vi "run.vi"(8 "error in (no error)":errorcluster, 11 "DL090324Microscope in":refnum<class "InstrumentDL090324.lvclass">) -> (0 "error out":errorcluster, 3 "DL090324Microscope out":refnum<class "InstrumentDL090324.lvclass">)   [LabVIEW 2010, in "InstrumentDL090324.lvclass"]
uses:
  InstrumentDL090324.lvclass
  internal_trigger_enum.ctl
  main/labview_source/controls/undock_button.ctl
  InstrumentDL090324.lvclass/InstrumentDL090324.ctl
  GenericInstrument/GenericInstrument/GenericInstrument.lvclass
  Detector/GenericDetector/GenericDetector/GenericDetector.lvclass
  LightSource/GenericLightSource/GenericLightSource/GenericLightSource.lvclass
  common/classes/ErrorController/ErrorController/class_data.vi
  common/classes/ErrorController/ErrorController/ErrorController.lvclass
panel:
  in  "button:undock":T1
  in  "Tab Control":enum32{"User", "Debug", "About"}(tab)
  in  "adjust buttons light source":bool[](array[boolean])
  in  "adjust buttons detectors":bool[](array[boolean])
  out "last trigger":T2
  out "statechart\nerror":errorcluster
  out "finished?":bool
  out "stache machine counter":i32
  # "Detectors"
  # "Light source"
  # "InstrumentDL090324\n\nImplemented by:\n- Dominik Langer, University of Zurich, Switzerland\n- Marcel van 't Hoff, University of Zurich, Switzerland"
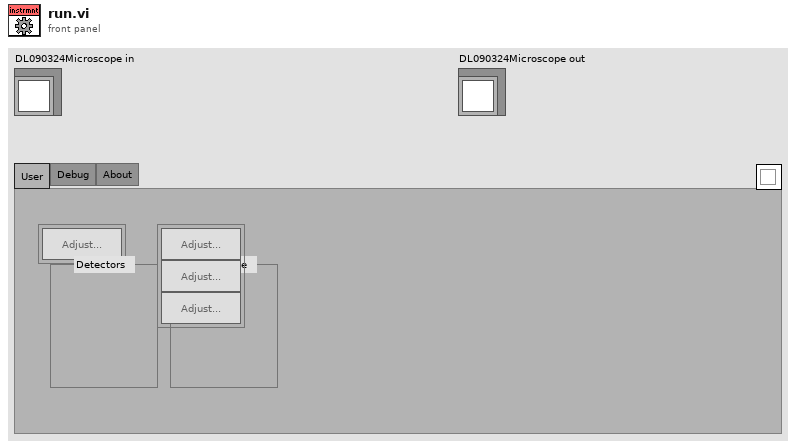
[diagram p1: front panel]
types:
  T1 = typedef "undock_button.ctl" = bool
  T2 = typedef "InstrumentDL090324.lvclass/internal_trigger_enum.ctl" = enum16{"NULL", "initialise", "terminate", "start", "stop"}
  T3 = typedef "top-level_component_type_enum.ctl" = enum16{"undefined", "ImagingMode", "ScanHead", "DAQ", "ImageAssembler", "Display", "DataCollection", "Analyser", "Stimulator", "ExperimentController", "Instrument", "Stage"}
  T4 = typedef "main_trigger_enum.ctl" = enum16{"NULL", "initialise", "terminate", "start", "stop", "change objective", "change experimentController", "change imagingMode", "save notebook", "started saving", "finished saving", "expCtr ready", "expCtr missing", "imgMd ready", "imgMd missing", "scanHd ready", "scanHd missing", "DAQ ready", "DAQ missing", "imgAsm ready", "imgAsm missing", "dataColl ready", "dataColl missing", "display ready", "display missing", "analysr ready", "analysr missing", "instrmnt ready", "instrmnt missing", "stimltr ready", "stimltr missing", "stage ready", "stage missing"}
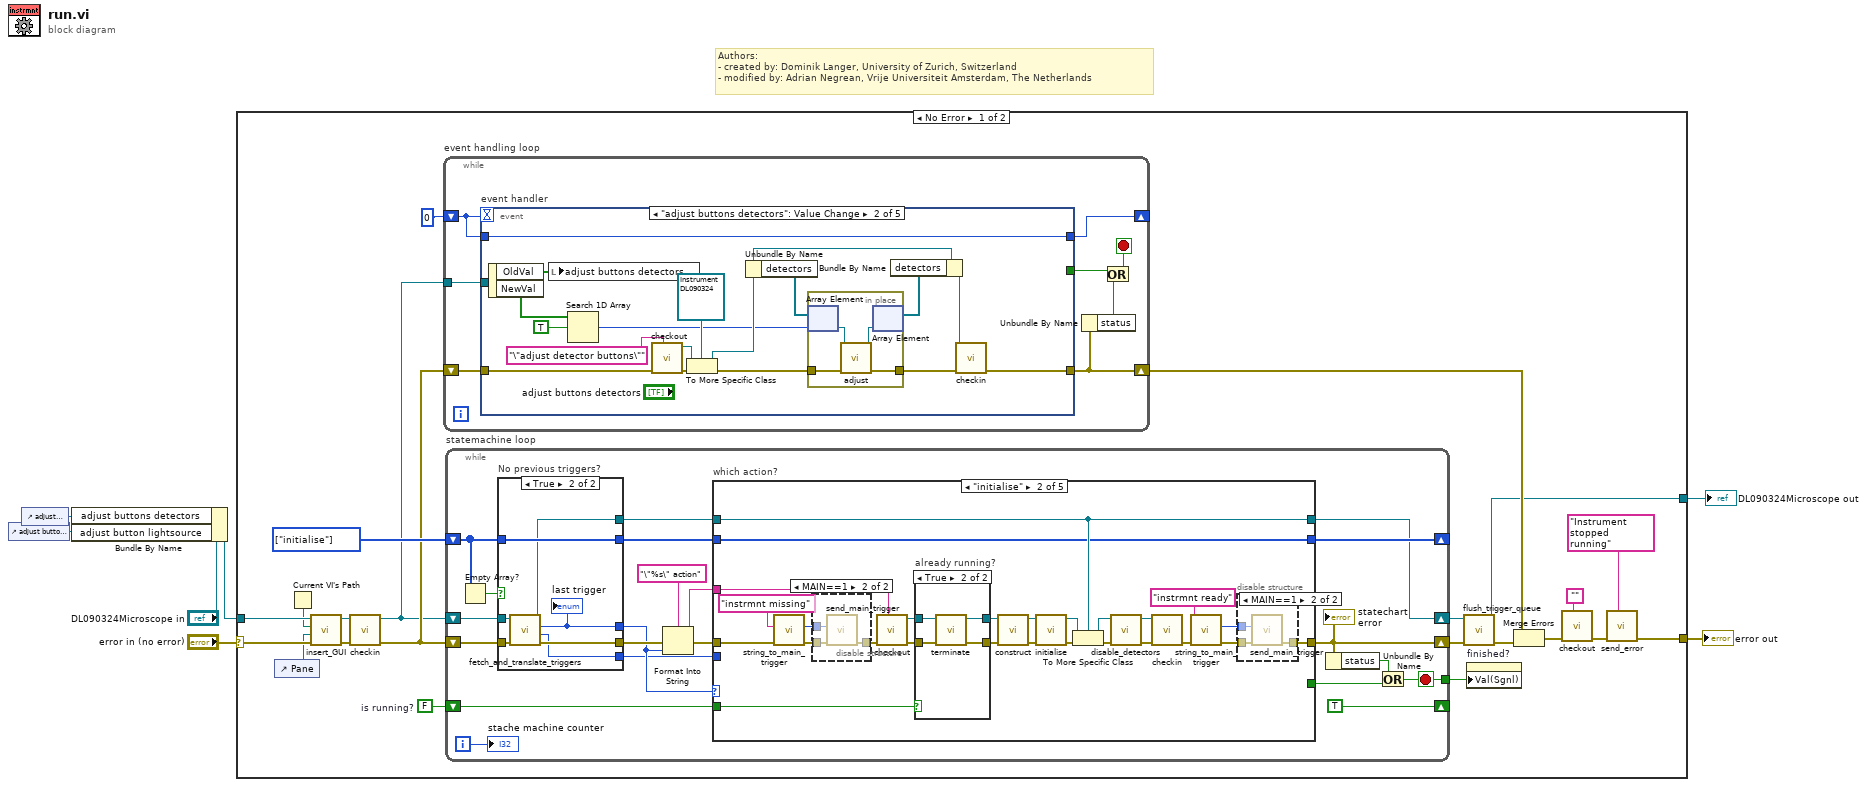
[diagram p0: block diagram]
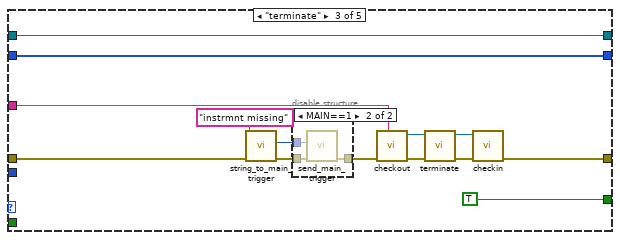
[diagram p6: hidden frame]
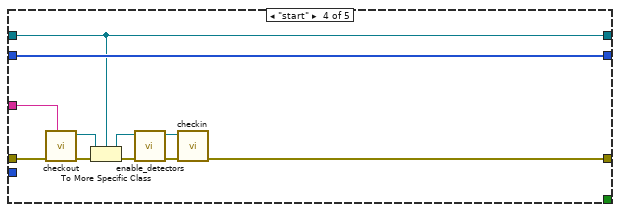
[diagram p8: hidden frame]
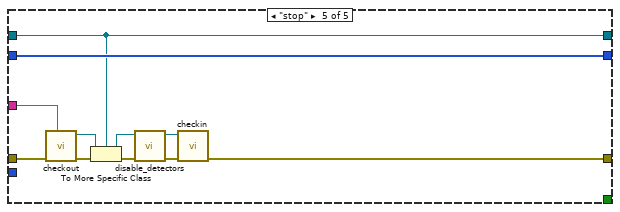
[diagram p9: hidden frame]
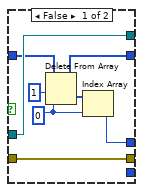
[diagram p10: hidden frame]
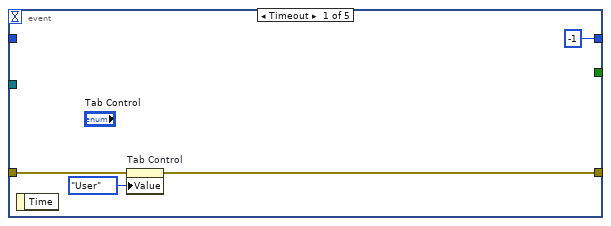
[diagram p11: hidden frame]
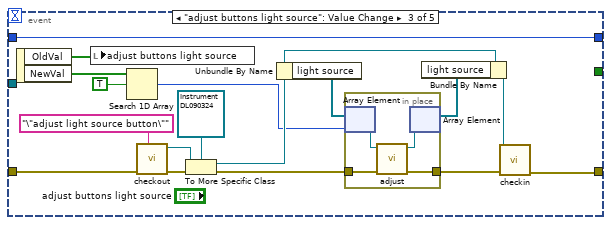
[diagram p12: hidden frame]
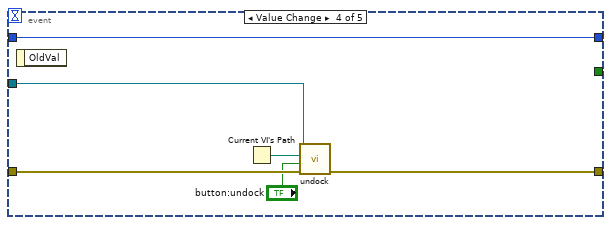
[diagram p13: hidden frame]
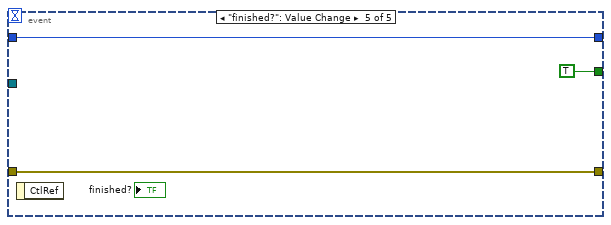
[diagram p14: hidden frame]
diagram:
  # "Authors: \n- created by: Dominik Langer, University of Zurich, Switzerland\n- modified by: Adrian Negrean, Vrije Universiteit Amsterdam, The Netherlands"
  n1 = control-ref of="adjust button lightsource"() -> (w1:refnum<vi>)
  n2 = control-ref of="adjust buttons detectors"() -> (w4:refnum<vi>)
  n3 = Bundle By Name(cluster="DL090324Microscope in", "adjust buttons detectors"=w4, "adjust button lightsource"=w1) -> (w2:refnum<class "InstrumentDL090324.lvclass">)
  n4 = case shown="No Error" "error in (no error)" {
    selector: "error in (no error)" -> [w27 w213]
    tunnel: [w22 w213] -> w6
    tunnel: [w12 w212] -> w5
    tunnel: w2 -> [w26 w212]
    frame No Error {
      w17 = FALSE  # is running?
      w18 = T2[] [enum."initialise"] items=["NULL", "initialise", "terminate", "start", "stop"]
      n5 = control-ref of="Pane"() -> (w24:refnum<vi>)
      n6 = Current VI's Path() -> (path=w25:path)
      n7 = call-dynamic "insert_GUI.vi"("error in (no error)"=w27, "Pane"=w24, "VI path"=w25, "GenericComponent in"=w26) -> ("error out"=w11:errorcluster, "GenericComponent out"=w19:refnum<class "InstrumentDL090324.lvclass">)  [unwired: 6 in]
      n8 = call-dynamic "checkin.vi"("error in (no error)"=w11, "GenericMicroscope in"=w19) -> ("error out"=w9:errorcluster, "GenericMicroscope out"=w8:refnum<class "InstrumentDL090324.lvclass">)  [unwired: 8 in]
      n9 = while "event handling loop" {
        shift-right: [w155] -> _
        shift-left: 0 -> [w156]
        shift-right: [w153] -> w13
        shift-left: w9 -> [w154]
        tunnel: w8 -> [w149]
        stop <- w152 stop-if-true
        n10 = event "event handler" shown="[1] \"adjust buttons detectors\": Value Change" {
          selector: _ -> [_ _ _ _ _]
          dyn-events: _ -> [_ _ _ _ _]
          timeout: w156 -> [_ _ _ _ _]
          tunnel: w156 -> [_ w177 w198 w208 w211]
          tunnel: [-1 w177 w198 w208 w211] -> w155
          tunnel: w154 -> [w158 w164 w197 w206 w210]
          tunnel: [w157 w172 w184 w205 w210] -> w153
          tunnel: [_ _ _ _ TRUE] -> w151
          tunnel: w149 -> [_ _ _ w207 _]
          event Timeout {
            n11 = event-data() -> ()  [unwired: 2 out]
            n12 = property on="Tab Control" class="TabCtl (strict)"(error in=w158, "Value"=enum32{"User", "Debug", "About"}."User" ("Tab Control")) -> (error out=w157:errorcluster)  [unwired: 1 in, 1 out]
          }
          event "adjust buttons detectors": Value Change {
            n13 = event-data() -> ("OldVal"=w175:bool[], "NewVal"=w169:bool[])  [unwired: 1 out]
            n14 = local write "adjust buttons detectors"(w175) -> ()
            n15 = Search 1D Array(1D array=w169, element=TRUE) -> (index of element=w167:i32)  [unwired: 1 out]
            n16 = call "checkout.vi"("locked by?"="\"adjust detector buttons\"", "error in (no error)"=w164) -> ("error out"=w161:errorcluster, "GenericMicroscope out"=w162:refnum<class "GenericInstrument.lvclass">)  [unwired: 8 out]
            n17 = To More Specific Class(target class=refnum<class "InstrumentDL090324.lvclass"> refnum ("DL090324Microscope.lvclass"), reference=w162, error in=w161) -> (specific class reference=w170:refnum<class "InstrumentDL090324.lvclass">, error out=w174:errorcluster)
            n18 = Unbundle By Name(w170) -> ("detectors"=w166:refnum<class "GenericDetector.lvclass">[])
            n19 = in-place {
              in-place-border: w174 -> [w181]
              in-place-border: [w178] -> w173
              n20 = in-place-array #1(w166, w167) -> (w180:refnum<class "GenericDetector.lvclass">)
              n21 = call-dynamic "adjust.vi"("error in (no error)"=w181, "GenericEmissionSensor in"=w180) -> ("error out"=w178:errorcluster, "GenericEmissionSensor out"=w179:refnum<class "GenericDetector.lvclass">)  [unwired: 8 out]
              n22 = in-place-array #1(w179) -> (w165:refnum<class "GenericDetector.lvclass">[])  [unwired: 1 out]
            }
            n23 = Bundle By Name(cluster=w170, "detectors"=w165) -> (w171:refnum<class "InstrumentDL090324.lvclass">)
            n24 = call-dynamic "checkin.vi"("error in (no error)"=w173, "GenericMicroscope in"=w171) -> ("error out"=w172:errorcluster)  [unwired: 8 in, 1 out]
          }
          event "adjust buttons light source": Value Change {
            n25 = event-data() -> ("OldVal"=w192:bool[], "NewVal"=w190:bool[])  [unwired: 1 out]
            n26 = local write "adjust buttons light source"(w192) -> ()
            n27 = Search 1D Array(1D array=w190, element=TRUE) -> (index of element=w182:i32)  [unwired: 1 out]
            n28 = call "checkout.vi"("locked by?"="\"adjust light source button\"", "error in (no error)"=w197) -> ("error out"=w196:errorcluster, "GenericMicroscope out"=w195:refnum<class "GenericInstrument.lvclass">)  [unwired: 8 out]
            n29 = To More Specific Class(target class=refnum<class "InstrumentDL090324.lvclass"> refnum ("DL090324Microscope.lvclass"), reference=w195, error in=w196) -> (specific class reference=w183:refnum<class "InstrumentDL090324.lvclass">, error out=w185:errorcluster)
            n30 = Unbundle By Name(w183) -> ("light source"=w187:refnum<class "GenericLightSource.lvclass">[])
            n31 = in-place {
              in-place-border: w185 -> [w202]
              in-place-border: [w201] -> w189
              n32 = in-place-array #2(w187, w182) -> (w200:refnum<class "GenericLightSource.lvclass">)
              n33 = call-dynamic "adjust.vi"("error in (no error)"=w202, "GenericLightSource in"=w200) -> ("error out"=w201:errorcluster, "GenericLightSource out"=w199:refnum<class "GenericLightSource.lvclass">)  [unwired: 8 in]
              n34 = in-place-array #2(w199) -> (w186:refnum<class "GenericLightSource.lvclass">[])  [unwired: 1 out]
            }
            n35 = Bundle By Name(cluster=w183, "light source"=w186) -> (w188:refnum<class "InstrumentDL090324.lvclass">)
            n36 = call-dynamic "checkin.vi"("error in (no error)"=w189, "GenericMicroscope in"=w188) -> ("error out"=w184:errorcluster)  [unwired: 8 in, 1 out]
          }
          event Value Change {
            n37 = event-data() -> ()  [unwired: 2 out]
            n38 = Current VI's Path() -> (path=w203:path)
            n39 = call-dynamic "undock.vi"("error in (no error)"=w206, "undock?"="button:undock", "VI path"=w203, "component in"=w207) -> ("error out"=w205:errorcluster)  [unwired: 6 in, 1 out]
          }
          event "finished?": Value Change {
            n40 = event-data() -> ()  [unwired: 2 out]
          }
        }
        n41 = Unbundle By Name(w153) -> ("status"=w150:bool)
        n42 = Or(x=w151, y=w150) -> (x .or. y?=w152:bool)
      }
      n43 = while "statemachine loop" {
        shift-right: [w34] -> w15
        shift-left: w9 -> [w50]
        shift-right: [w40] -> _
        shift-left: w18 -> [w48]
        shift-right: [w38] -> w14
        shift-left: w8 -> [w49]
        shift-right: [TRUE ("is running?")] -> _
        shift-left: w17 -> [w37]
        tunnel: [w31] -> w16
        i -> [w30]
        stop <- w31 stop-if-true
        n44 = Empty Array?(array=w48) -> (empty?=w47:bool)
        n45 = case "No previous triggers?" shown="True" w47 {
          tunnel: w49 -> [w141 w145]
          tunnel: w50 -> [w139 w147]
          tunnel: [w141 w144] -> w39
          tunnel: [w137 w143] -> w44
          tunnel: [_ w142] -> w43
          tunnel: [w139 w146] -> w46
          tunnel: w48 -> [w140 w148]
          tunnel: [w136 w148] -> w41
          frame False {
            w134 = 0 ("index")
            n46 = Delete From Array(array=w140, length=1, index=w134) -> (deleted portion=w138:T2[], array with subset deleted=w136:T2[])
            n47 = Index Array(array=w138, index=w134) -> (element=w137:T2)
          }
          frame True {
            n48 = call-dynamic "fetch_and_translate_triggers.vi"("error in (no error)"=w147, "InstrumentDL090324 in"=w145) -> ("error out"=w146:errorcluster, "sender TLC type"=w142:T3, "statechart trigger"=w143:T2, "InstrumentDL090324 out"=w144:refnum<class "InstrumentDL090324.lvclass">)  [unwired: 6 in]
            "last trigger" <- w143
          }
        }
        n49 = Format Into String(format string="\"%s\" action", error in=w46, w44) -> (resulting string=w35:string, error out=w42:errorcluster)  [unwired: 1 in]
        n50 = case "which action?" shown="\"initialise\"" w44 {
          tunnel: w43 -> [_ _ _ _ _]
          tunnel: w42 -> [w51 w56 w95 w121 w132]
          tunnel: w41 -> [w53 w63 w107 w122 w133]
          tunnel: [w53 w63 w107 w122 w133] -> w40
          tunnel: w39 -> [w52 w66 w106 w117 w128]
          tunnel: [w52 w66 w106 w117 w128] -> w38
          tunnel: [w51 w71 w103 w116 w127] -> w34
          tunnel: w37 -> [_ w79 _ _ _]
          tunnel: w35 -> [_ w76 w102 w120 w131]
          tunnel: [_ _ TRUE ("is running?") _ _] -> w32
          frame "NULL", Default {
          }
          frame "initialise" {
            n51 = call "string_to_main_trigger.vi"("error in (no error)"=w56, "trigger string"="instrmnt missing") -> ("error out"=w57:errorcluster, "main trigger"=w58:T4)  [unwired: 8 in]
            n52 = disable-structure shown="MAIN==1" {
              disable-tunnel: [w80 w82] -> w55
              disable-tunnel: w57 -> [w80 w83]
              disable-tunnel: w58 -> [_ w81]
              frame condition #0 (active) {
              }
              frame condition #1 {
                n53 = call "send_main_trigger.vi"("error in (no error)"=w83, "trigger"=w81) -> ("error out"=w82:errorcluster)  [unwired: 9 in]
              }
            }
            n54 = call "checkout.vi"("locked by?"=w76, "error in (no error)"=w55) -> ("error out"=w78:errorcluster, "GenericMicroscope out"=w77:refnum<class "GenericInstrument.lvclass">)  [unwired: 8 out]
            n55 = case "already running?" shown="True" w79 {
              tunnel: w78 -> [w88 w93]
              tunnel: w77 -> [w89 w91]
              tunnel: [w88 w92] -> w75
              tunnel: [w89 w90] -> w74
              frame False {
              }
              frame True {
                n56 = call-dynamic "terminate.vi"("error in (no error)"=w93, "GenericPlugin in"=w91) -> ("error out"=w92:errorcluster, "GenericPlugin out"=w90:refnum<class "GenericInstrument.lvclass">)  [unwired: 8 out]
              }
            }
            n57 = call-dynamic "construct.vi"("error in (no error)"=w75, "GenericPlugin in"=w74) -> ("error out"=w72:errorcluster, "GenericPlugin out"=w73:refnum<class "GenericInstrument.lvclass">)  [unwired: 2 in, 6 out]
            n58 = call-dynamic "initialise.vi"("error in (no error)"=w72, "GenericPlugin in"=w73) -> ("error out"=w68:errorcluster, "GenericPlugin out"=w65:refnum<class "GenericInstrument.lvclass">)  [unwired: 8 in]
            n59 = To More Specific Class(target class=w66, reference=w65, error in=w68) -> (specific class reference=w64:refnum<class "InstrumentDL090324.lvclass">, error out=w67:errorcluster)
            n60 = call-dynamic "disable_detectors.vi"("error in (no error)"=w67, "DL090324Microscope in"=w64) -> ("error out"=w70:errorcluster, "DL090324Microscope out"=w69:refnum<class "InstrumentDL090324.lvclass">)  [unwired: 8 out]
            n61 = call-dynamic "checkin.vi"("error in (no error)"=w70, "GenericMicroscope in"=w69) -> ("error out"=w61:errorcluster)  [unwired: 8 in, 1 out]
            n62 = call "string_to_main_trigger.vi"("error in (no error)"=w61, "trigger string"="instrmnt ready") -> ("error out"=w60:errorcluster, "main trigger"=w59:T4)  [unwired: 8 in]
            n63 = disable-structure shown="MAIN==1" {
              disable-tunnel: [w84 w86] -> w71
              disable-tunnel: w60 -> [w84 w87]
              disable-tunnel: w59 -> [_ w85]
              frame condition #0 (active) {
              }
              frame condition #1 {
                n64 = call "send_main_trigger.vi"("error in (no error)"=w87, "trigger"=w85) -> ("error out"=w86:errorcluster)  [unwired: 9 in]
              }
            }
          }
          frame "terminate" {
            n65 = call "string_to_main_trigger.vi"("error in (no error)"=w95, "trigger string"="instrmnt missing") -> ("error out"=w97:errorcluster, "main trigger"=w96:T4)  [unwired: 8 in]
            n66 = disable-structure shown="MAIN==1" {
              disable-tunnel: [w108 w110] -> w94
              disable-tunnel: w97 -> [w108 w111]
              disable-tunnel: w96 -> [_ w109]
              frame condition #0 (active) {
              }
              frame condition #1 {
                n67 = call "send_main_trigger.vi"("error in (no error)"=w111, "trigger"=w109) -> ("error out"=w110:errorcluster)  [unwired: 9 in]
              }
            }
            n68 = call "checkout.vi"("locked by?"=w102, "error in (no error)"=w94) -> ("error out"=w105:errorcluster, "GenericMicroscope out"=w101:refnum<class "GenericInstrument.lvclass">)  [unwired: 8 out]
            n69 = call-dynamic "terminate.vi"("error in (no error)"=w105, "GenericPlugin in"=w101) -> ("error out"=w104:errorcluster, "GenericPlugin out"=w100:refnum<class "GenericInstrument.lvclass">)  [unwired: 8 out]
            n70 = call-dynamic "checkin.vi"("error in (no error)"=w104, "GenericMicroscope in"=w100) -> ("error out"=w103:errorcluster)  [unwired: 8 in, 1 out]
          }
          frame "start" {
            n71 = call "checkout.vi"("locked by?"=w120, "error in (no error)"=w121) -> ("error out"=w119:errorcluster, "GenericMicroscope out"=w118:refnum<class "GenericInstrument.lvclass">)  [unwired: 8 out]
            n72 = To More Specific Class(target class=w117, reference=w118, error in=w119) -> (specific class reference=w115:refnum<class "InstrumentDL090324.lvclass">, error out=w113:errorcluster)
            n73 = call-dynamic "enable_detectors.vi"("error in (no error)"=w113, "DL090324Microscope in"=w115) -> ("error out"=w112:errorcluster, "DL090324Microscope out"=w114:refnum<class "InstrumentDL090324.lvclass">)  [unwired: 8 out]
            n74 = call-dynamic "checkin.vi"("error in (no error)"=w112, "GenericMicroscope in"=w114) -> ("error out"=w116:errorcluster)  [unwired: 8 in, 1 out]
          }
          frame "stop" {
            n75 = call "checkout.vi"("locked by?"=w131, "error in (no error)"=w132) -> ("error out"=w130:errorcluster, "GenericMicroscope out"=w129:refnum<class "GenericInstrument.lvclass">)  [unwired: 8 out]
            n76 = To More Specific Class(target class=w128, reference=w129, error in=w130) -> (specific class reference=w126:refnum<class "InstrumentDL090324.lvclass">, error out=w124:errorcluster)
            n77 = call-dynamic "disable_detectors.vi"("error in (no error)"=w124, "DL090324Microscope in"=w126) -> ("error out"=w123:errorcluster, "DL090324Microscope out"=w125:refnum<class "InstrumentDL090324.lvclass">)  [unwired: 8 out]
            n78 = call-dynamic "checkin.vi"("error in (no error)"=w123, "GenericMicroscope in"=w125) -> ("error out"=w127:errorcluster)  [unwired: 8 in, 1 out]
          }
        }
        "statechart\nerror" <- w34
        n79 = Unbundle By Name(w34) -> ("status"=w33:bool)
        n80 = Or(x=w33, y=w32) -> (x .or. y?=w31:bool)
        "stache machine counter" <- w30
      }
      n81 = call-dynamic "flush_trigger_queue.vi"("error in (no error)"=w15, "GenericToplevelComponent in"=w14) -> ("error out"=w10:errorcluster, "GenericToplevelComponent out"=w12:refnum<class "InstrumentDL090324.lvclass">)  [unwired: 8 in]
      n82 = property on="finished?" class="Bool (strict)"("Val(Sgnl)"=w16) -> ()  [unwired: 2 in, 2 out]
      n83 = Merge Errors(w13, w10) -> (w20:errorcluster)
      n84 = call "checkout.vi"("locked by?"="", "error in (no error)"=w20) -> ("error out"=w23:errorcluster)  [unwired: 9 out]
      n85 = call "send_error.vi"("additional message"="Instrument stopped running", "error in (no error)"=w23) -> ("error out"=w22:errorcluster)  [unwired: 9 in]
    }
    frame Error {
    }
  }
  "error out" <- w6
  "DL090324Microscope out" <- w5
